vi "ClientPool_CreateDestroyAndRecreateClients_ClientsCreatedWithNonZeroGrpcId.vi"(8 "error in (no error)":errorcluster) -> (0 "error out":errorcluster, 2 "result":string, 3 "pass":bool)   [LabVIEW 2020, in "MeasurementServerTests.lvlib"]
uses:
  MeasurementServerTests.lvlib
  Runtime/MeasurementLink gRPC Utilities/GrpcClientPool/gRPC Client Pool.lvclass
  Runtime/MeasurementLink gRPC Utilities/GrpcClientPool/FGV Action.ctl
panel:
  in  "Action":T1
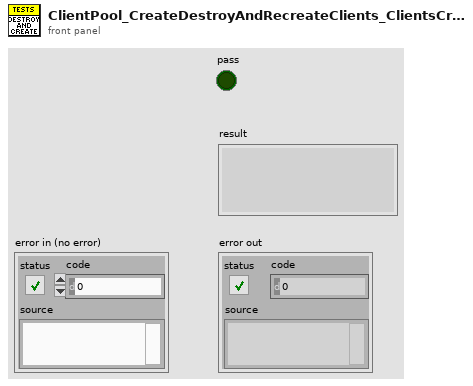
[diagram p1: front panel]
types:
  T1 = typedef "gRPC Utilities.lvlib/gRPC Client Pool.lvclass/FGV Action.ctl" = enum16{"Get Discovery Client", "Get Session Client", "Get Pinmap Client", "Destroy Clients"}
  T2 = typedef "grpc-lvsupport-release.lvlib/grpcId.ctl" = u64
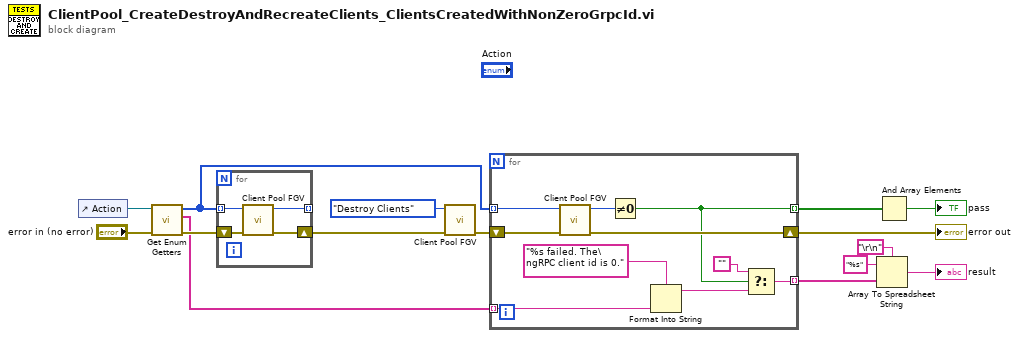
[diagram p0: block diagram]
diagram:
  n1 = control-ref of="Action"() -> (w14:refnum<vi>)
  n2 = call "Get Enum Getters.vi"("error in (no error)"="error in (no error)", "enum ref in"=w14) -> ("error out"=w13:errorcluster, "enum strings"=w2:string[], "enum numbers"=w1:i32[])  [unwired: 7 in]
  n3 = for {
    tunnel: w1 -> [w19] mode=indexing
    shift-right: [w17] -> w12
    shift-left: w13 -> [w18]
    tunnel: [w16] -> _ mode=indexing
    n4 = call "Client Pool FGV.vi"("error in (no error)"=w18, "Action"=w19) -> ("error out"=w17:errorcluster, "grpc client id"=w16:T2)  [unwired: 8 in]
  }
  n5 = call "Client Pool FGV.vi"("error in (no error)"=w12, "Action"=FGV_Action."Destroy Clients") -> ("error out"=w3:errorcluster)  [unwired: 8 in, 1 out]
  n6 = for {
    shift-right: [w28] -> w5
    shift-left: w3 -> [w29]
    tunnel: w1 -> [w20] mode=indexing
    tunnel: [w25] -> w10 mode=indexing
    tunnel: w2 -> [w27] mode=indexing
    tunnel: [w22] -> w9 mode=indexing
    n7 = call "Client Pool FGV.vi"("error in (no error)"=w29, "Action"=w20) -> ("error out"=w28:errorcluster, "grpc client id"=w21:T2)  [unwired: 8 in]
    n8 = Not Equal To 0?(x=w21) -> (x != 0?=w25:bool)
    n9 = Format Into String(format string="%s failed. The\ngRPC client id is 0." ("result"), w27) -> (resulting string=w24:string)  [unwired: 2 in, 1 out]
    n10 = Select(t="", s=w25, f=w24) -> (s? t:f=w22:string)
  }
  "error out" <- w5
  n11 = Array To Spreadsheet String(delimiter (Tab)="\r\n", array=w9, 3:"%s" ("format string")) -> (spreadsheet string=→"result":string)
  n12 = And Array Elements(Boolean array=w10) -> (logical AND=→"pass":bool)
